vi "FpgaTest.vi"() -> ()   [LabVIEW 2020]
uses:
  <vilib>/rvi/Emulation/niFpgaGetClockAttributes.vi
  <vilib>/rvi/Emulation/niFpgaSctlEmulationGetInTimedLoop.vi
  <vilib>/rvi/Emulation/niFpgaEmulationReportErrorSimple.vi
  <vilib>/rvi/Emulation/niFpgaCriticalErrorInLSC.vi
panel:
  in  "U64ArrayIn":u64[](array[numeric])=[0, 0, 0, 0, 0, 0, 0, 0]
  out "U64ArrayOut":u64[](array[numeric])
  out "I16ArrayOut":i16[](array[numeric])
  in  "I16ArrayIn":i16[](array[numeric])=[0, 0, 0, 0, 0, 0, 0, 0]
  in  "U64In":u64
  in  "U32In":u32
  in  "U16In":u16
  in  "U8In":u8
  in  "I64In":i64
  in  "I32In":i32
  in  "I16In":i16
  in  "I8In":i8
  out "BoolOut":bool
  in  "BoolIn":bool
  out "U64Out":u64
  out "U32Out":u32
  out "U16Out":u16
  out "I64Out":i64
  out "I32Out":i32
  out "I8Out":i8
  out "U8Out":u8
  out "I16":i16
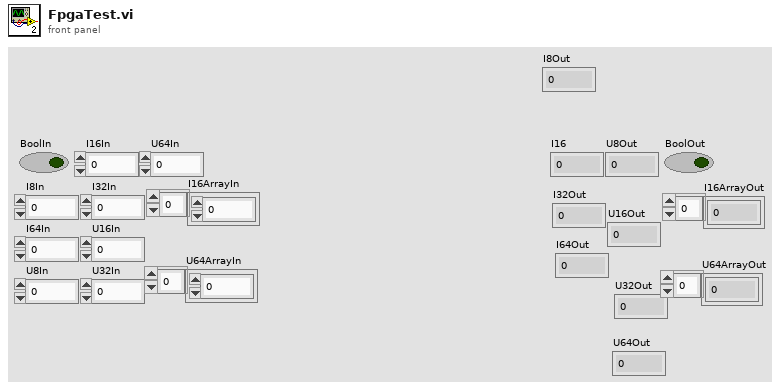
[diagram p1: front panel]
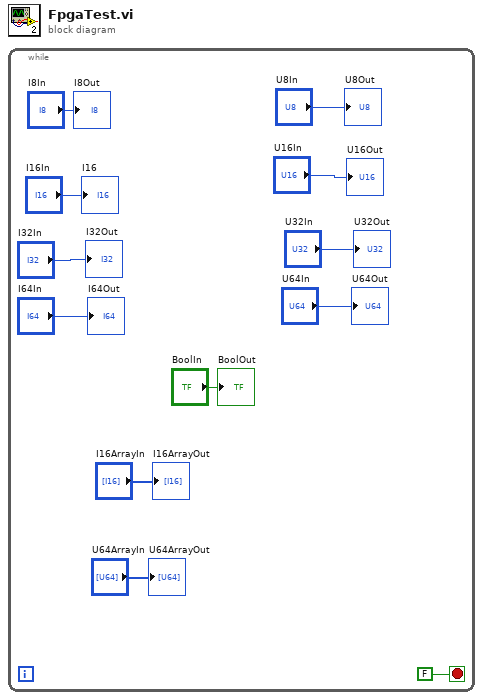
[diagram p0: block diagram]
diagram:
  n1 = while {
    stop <- FALSE stop-if-true
    "I16" <- "I16In"
    "U8Out" <- "U8In"
    "I8Out" <- "I8In"
    "I32Out" <- "I32In"
    "I64Out" <- "I64In"
    "U16Out" <- "U16In"
    "U32Out" <- "U32In"
    "U64Out" <- "U64In"
    "BoolOut" <- "BoolIn"
    "I16ArrayOut" <- "I16ArrayIn"
    "U64ArrayOut" <- "U64ArrayIn"
  }
